vi "Grow primitive into new lattice vectors.vi"(6 "Max # of atoms":i32=9999999, 7 "Keep old lattice vectors?":bool, 8 "New Lattice Vector c":dbl[](array[numeric])=[0.0, 0.0, 6.0], 9 "New Lattice Vector b":dbl[](array[numeric])=[0.0, 6.0, 0.0], 10 "New Lattice Vector a":dbl[](array[numeric])=[6.0, 0.0, 0.0], 11 "Primitive":T1={"Structure Name"="Gamm8 Subcrystal", "Lattice vector a"=[2.3379684769090283, 4.050155798593294, -3.073453095936429e-05], "Lattice vector b"=[0.0, 2.7000749366574968, 3.8175198422845327], "Lattice vector c"=[4.675927601962877, 0.0, 0.0], "Atoms Array"=[{"Atom Name"="Cd", "Positions (Direct)"=[[0.0, 2.2797955771e-06, 0.2499966378910753]], "Positions (Cartesian)"=[[0.0, -3.2294507389786483e-06, 2.863111017657439]]}, {"Atom Name"="Te", "Positions (Direct)"=[[0.0, -2.2797955771e-06, 3.3621089247e-06]], "Positions (Cartesian)"=[[0.0, -1.5237858666867705e-05, -2.8630725126350507]]}], "# of atoms"=2} {"Atoms Array"."Positions (Cartesian)" format="%#_4f"; "Atoms Array"."Positions (Direct)" format="%#_4f"}) -> (0 "error out":errorcluster, 2 "Supercells Filled":dbl[][](array[numeric]), 3 "Expanded to new Vectors":T1={"Structure Name"="Gamm8 Subcrystal", "Lattice vector a"=[2.3379684769090283, 4.050155798593294, -3.073453095936429e-05], "Lattice vector b"=[0.0, 2.7000749366574968, 3.8175198422845327], "Lattice vector c"=[4.675927601962877, 0.0, 0.0], "Atoms Array"=[{"Atom Name"="Cd", "Positions (Direct)"=[[0.0, 2.2797955771e-06, 0.2499966378910753]], "Positions (Cartesian)"=[[0.0, -3.2294507389786483e-06, 2.863111017657439]]}, {"Atom Name"="Te", "Positions (Direct)"=[[0.0, -2.2797955771e-06, 3.3621089247e-06]], "Positions (Cartesian)"=[[0.0, -1.5237858666867705e-05, -2.8630725126350507]]}], "# of atoms"=2} {"Atoms Array"."Positions (Cartesian)" format="%#_4f"; "Atoms Array"."Positions (Direct)" format="%#_4f"})   [LabVIEW 2010]
uses:
  <vilib>/Analysis/baseanly.llb/Real Inverse Matrix.vi
  <vilib>/Analysis/baseanly.llb/A x Vector.vi
  <vilib>/Analysis/NI_AALBase.lvlib
panel:
  out "Numeric 2":i32
  out "Numeric":i32
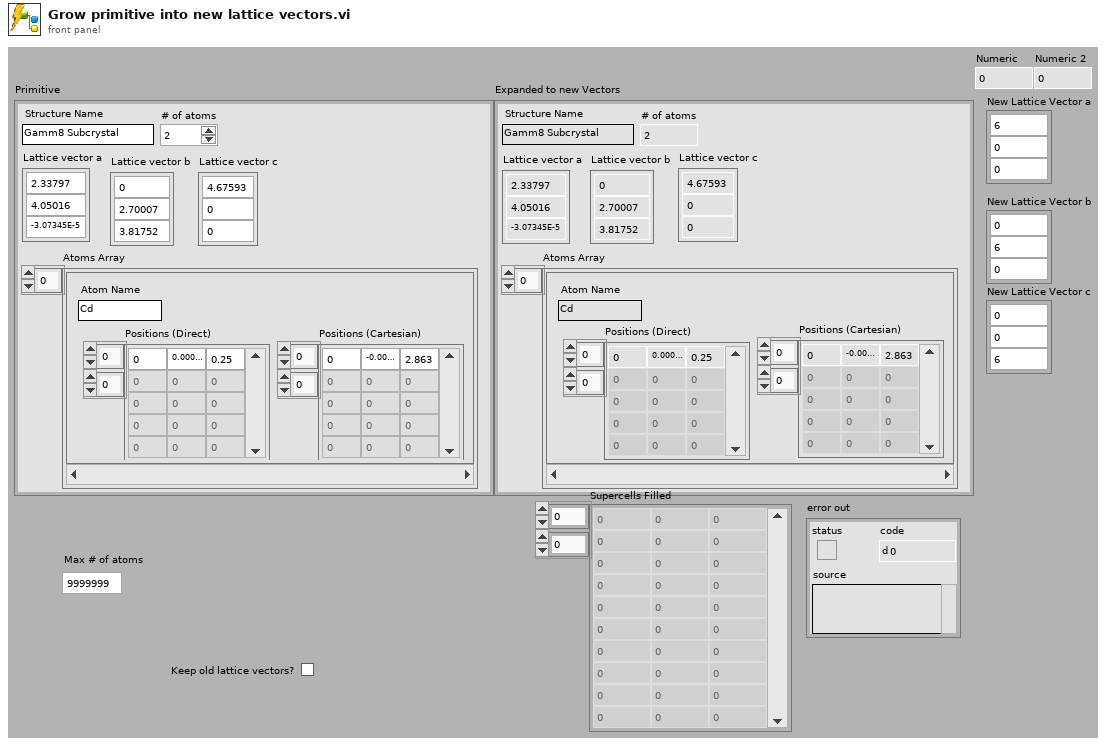
[diagram p1: front panel]
types:
  T1 = cluster{"Structure Name":string, "Lattice vector a":dbl[], "Lattice vector b":dbl[], "Lattice vector c":dbl[], "Atoms Array":cluster{"Atom Name":string, "Positions (Direct)":dbl[][], "Positions (Cartesian)":dbl[][]}[], "# of atoms":i32}
  T2 = cluster{"Atom Name":string, "Positions (Direct)":dbl[][], "Positions (Cartesian)":dbl[][]}[]
  T3 = typedef "NI_Matrix.lvlib/RealMatrix.ctl" = dbl[][]
  T4 = cluster{"Atom Name":string, "Positions (Direct)":dbl[][], "Output Array":dbl[][]}
  T5 = cluster{string, "Lattice vector a":dbl[], "Lattice vector b":dbl[], "Lattice vector c":dbl[], cluster{"Atom Name":string, "Positions (Direct)":dbl[][], "Output Array":dbl[][]}[], i32}
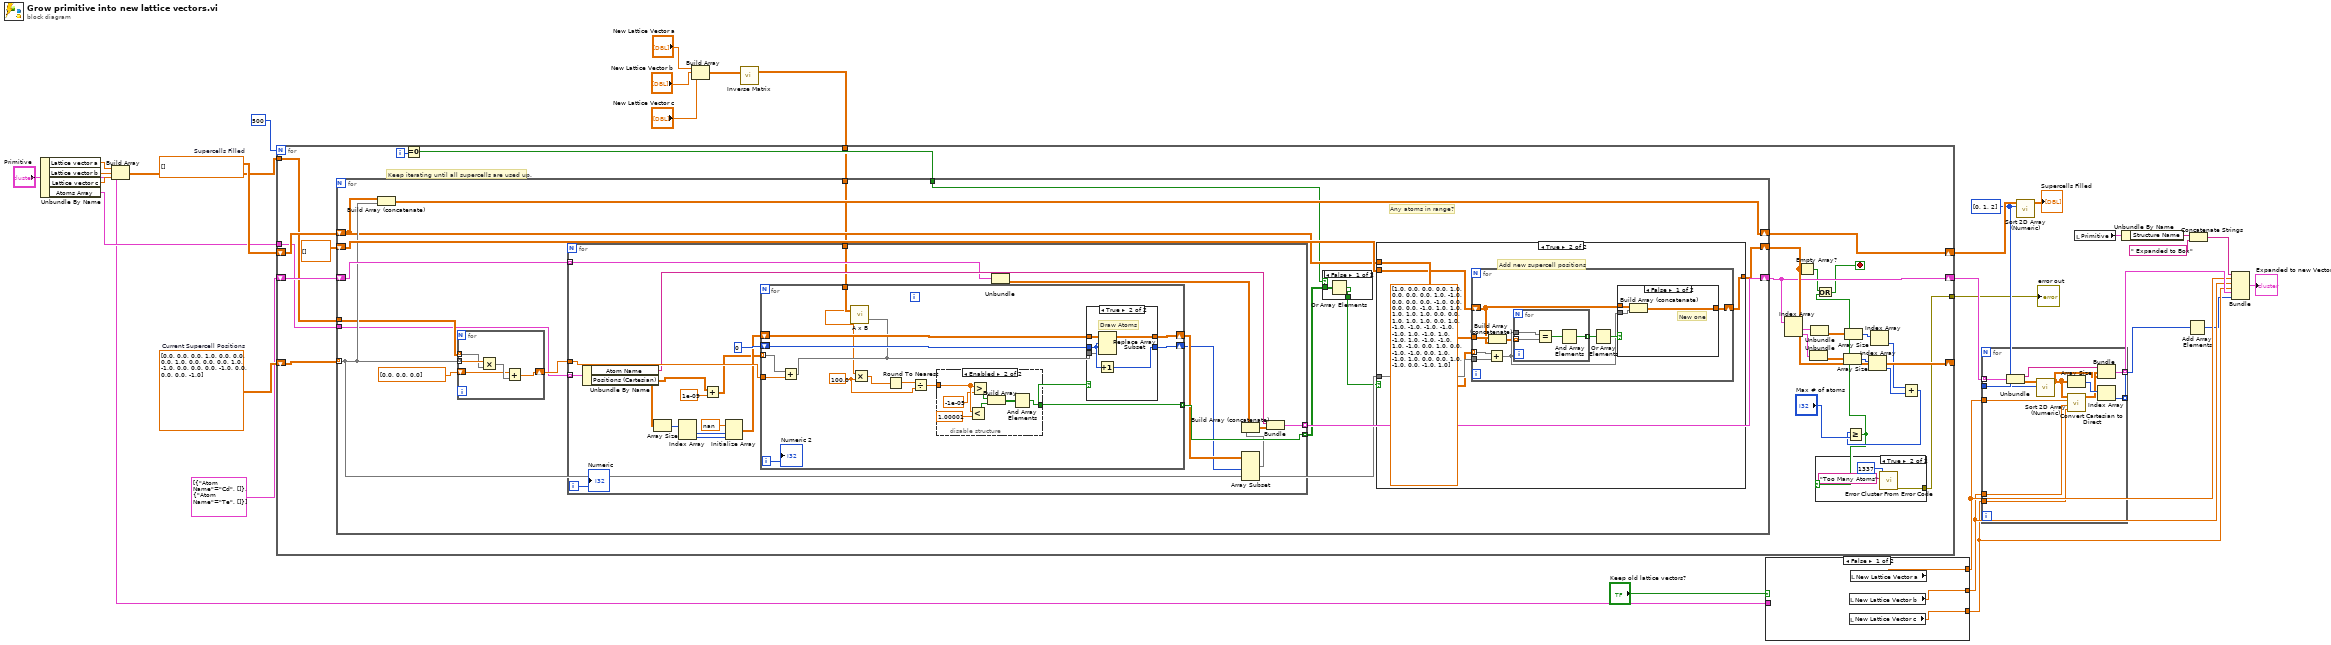
[diagram p0: block diagram]
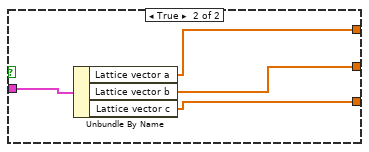
[diagram p2: hidden frame]
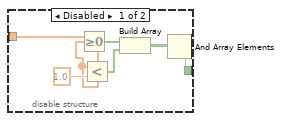
[diagram p7: hidden frame]
diagram:
  w20 = i32[] [0, 1, 2] ("Sort by Cols")
  w30 = dbl[][] []  # Supercells Filled
  w32 = dbl[][] [[0.0, 0.0, 0.0], [1.0, 0.0, 0.0], [0.0, 1.0, 0.0], [0.0, 0.0, 1.0], [-1.0, 0.0, 0.0], [0.0, -1.0, 0.0], [0.0, 0.0, -1.0]]  # Current Supercell Positions
  n1 = Unbundle By Name("Primitive") -> ("Lattice vector a"=w29:dbl[], "Lattice vector b"=w28:dbl[], "Lattice vector c"=w27:dbl[], "Atoms Array"=w25:T2)
  n2 = Build Array(w29, w28, w27) -> (w26:dbl[][])
  n3 = Build Array("New Lattice Vector a", "New Lattice Vector b", "New Lattice Vector c") -> (w2:T3)
  n4 = call-poly <vilib>:"Inverse Matrix.vi"("Input Matrix"=w2) -> ("Inverse Matrix"=w1:T3)  [unwired: 1 in, 1 out]
  n5 = for {
    N: 500 -> [_]
    shift-right: [w52] -> _
    shift-left: w32 -> [w33]
    shift-right: [w49] -> w21
    shift-left: cluster{"Atom Name":string, dbl[][]}[] [{"Atom Name"="Cd", []}, {"Atom Name"="Te", []}] -> [w57]
    shift-right: [w55] -> w24
    shift-left: w30 -> [w56]
    tunnel: w26 -> [w54]
    tunnel: w25 -> [w53]
    tunnel: [w35] -> w6
    tunnel: w1 -> [w34]
    i -> [w51]
    stop <- w44 stop-if-true
    # "Keep iterating until all supercells are used up."
    n6 = Equal To 0?(x=w51) -> (x = 0?=w50:bool)
    n7 = for {
      shift-right: [w71] -> w52
      shift-left: dbl[][] [] ("Supercell Positions") -> [w74]
      tunnel: w33 -> [w70] mode=indexing
      shift-right: [w73] -> w49
      shift-left: w57 -> [w72]
      shift-right: [w66] -> w55
      shift-left: w56 -> [w69]
      tunnel: w54 -> [w68]
      tunnel: w53 -> [w67]
      tunnel: w50 -> [w63]
      tunnel: w34 -> [w62]
      # "Any atoms in range?"
      n8 = Build Array (concatenate)(w69, w70) -> (w66:dbl[][])
      n9 = for {
        tunnel: w70 -> [w107] mode=indexing
        shift-right: [w105] -> w75
        shift-left: dbl[] [0.0, 0.0, 0.0] -> [w104]
        tunnel: w68 -> [w103] mode=indexing
        n10 = Multiply(x=w107, y=w103) -> (x*y=w106:dbl[])
        n11 = Add(x=w104, y=w106) -> (x+y=w105:dbl[])
      }
      n12 = for {
        tunnel: w67 -> [w128] mode=indexing
        tunnel: w75 -> [w129]
        tunnel: [w127] -> w65 mode=indexing
        tunnel: w72 -> [w124] mode=indexing
        tunnel: [w125] -> w73 mode=indexing
        tunnel: w62 -> [w112]
        i -> [w108]
        n13 = Unbundle By Name(w128) -> ("Atom Name"=w126:string, "Positions (Cartesian)"=w110:dbl[][])
        n14 = Array Size(array=w110) -> (size(s)=w118:i32[])
        n15 = Index Array(array=w118) -> (element #1=w117:i32, element #2=w116:i32)  [unwired: 2 in]
        n16 = Add(x=w110, y=1e-09) -> (x+y=w109:dbl[][])
        n17 = Initialize Array(nan ("element"), w117, w116) -> (w119:dbl[][])
        n18 = for {
          tunnel: w109 -> [w144] mode=indexing
          tunnel: w129 -> [w143]
          shift-right: [w142] -> w115
          shift-left: w119 -> [w141]
          tunnel: [w137] -> w127 mode=indexing
          shift-right: [w139] -> w114
          shift-left: 0 -> [w140]
          tunnel: w112 -> [w138]
          i -> [w133]
          w134 = 100.0 ("y")
          n19 = Add(x=w144, y=w143) -> (x+y=w132:dbl[])
          n20 = call-poly <vilib>:"A x B.vi"("Vector"=w132, "A"=w138) -> ("A x Vector"=w131:dbl[])  [unwired: 1 out]
          n21 = Multiply(x=w131, y=w134) -> (x*y=w136:dbl[])
          n22 = Round To Nearest(number=w136) -> (nearest integer value=w135:dbl[])
          n23 = Divide(x=w135, y=w134) -> (x/y=w130:dbl[])
          n24 = disable-structure shown="Enabled" {
            disable-tunnel: [w146 w152] -> w137
            disable-tunnel: w130 -> [w145 w156]
            frame Disabled {
              n25 = Greater Or Equal To 0?(x=w145) -> (x >= 0?=w149:bool[])
              n26 = Less?(x=w145, y=1.0) -> (x < y?=w148:bool[])
              n27 = Build Array(w149, w148) -> (w147:bool[][])
              n28 = And Array Elements(Boolean array=w147) -> (logical AND=w146:bool)
            }
            frame Enabled {
              n29 = Less?(x=w156, y=1.00001) -> (x < y?=w154:bool[])
              n30 = Greater?(x=w156, y=-1e-05) -> (0:w153:bool[])
              n31 = Build Array(w153, w154) -> (w155:bool[][])
              n32 = And Array Elements(Boolean array=w155) -> (logical AND=w152:bool)
            }
          }
          n33 = case shown="True" w137 {
            tunnel: w132 -> [_ w161]
            tunnel: [w159 w160] -> w142
            tunnel: w141 -> [w159 w163]
            tunnel: w140 -> [w158 w162]
            tunnel: [w158 w164] -> w139
            frame False {
              # "Not inside box"
            }
            frame True {
              # "Draw Atoms"
              n34 = Increment(x=w162) -> (x+1=w164:i32)
              n35 = Replace Array Subset(array=w163, new element=w161, index (row)=w162) -> (w160:dbl[][])  [unwired: 1 in]
            }
          }
          "Numeric 2" <- w133
        }
        n36 = Unbundle(w124) -> (w122:dbl[][])  [unwired: 1 out]
        n37 = Array Subset(array=w115, length (row)=w114) -> (w113:dbl[][])  [unwired: 3 in]
        n38 = Build Array (concatenate)(w122, w113) -> (w121:dbl[][])
        n39 = Bundle("Atom Name"=w126, w121) -> (w125:cluster{"Atom Name":string, dbl[][]})  [unwired: 1 in]
        "Numeric" <- w108
      }
      n40 = case shown="False" w63 {
        selector: w63 -> [_ w79]
        tunnel: w65 -> [w78 _]
        tunnel: [w77 w79] -> w64
        frame False {
          n41 = Or Array Elements(Boolean array=w78) -> (logical OR=w77:bool)
        }
        frame True {
        }
      }
      n42 = case shown="True" w64 {
        tunnel: w70 -> [_ w85]
        tunnel: [w80 w81] -> w71
        tunnel: w74 -> [w80 w82]
        tunnel: w69 -> [_ w83]
        frame False {
          # "Don't sweat it"
        }
        frame True {
          # "Add new supercell positions"
          n43 = for {
            tunnel: w85 -> [w93]
            tunnel: dbl[][] [[1.0, 0.0, 0.0], [0.0, 1.0, 0.0], [0.0, 0.0, 1.0], [-1.0, 0.0, 0.0], [0.0, -1.0, 0.0], [0.0, 0.0, -1.0], [1.0, 1.0, 1.0], [1.0, 1.0, 0.0], [0.0, 1.0, 1.0], [1.0, 0.0, 1.0], [-1.0, -1.0, -1.0], [-1.0, -1.0, 1.0], [-1.0, 1.0, -1.0], [1.0, -1.0, -1.0], [1.0, -1.0, 0.0], [1.0, 0.0, -1.0], [-1.0, 0.0, 1.0], [-1.0, 1.0, 0.0], [0.0, 1.0, -1.0], [0.0, -1.0, 1.0]] -> [w94] mode=indexing
            tunnel: w83 -> [w88]
            shift-right: [w92] -> w81
            shift-left: w82 -> [w87]
            n44 = Add(x=w94, y=w93) -> (x+y=w90:dbl[])
            n45 = Build Array (concatenate)(w88, w87) -> (w86:dbl[][])
            n46 = for {
              tunnel: w90 -> [w102]
              tunnel: w86 -> [w101] mode=indexing
              tunnel: [w99] -> w89 mode=indexing
              n47 = Equal?(x=w102, y=w101) -> (x = y?=w100:bool[])
              n48 = And Array Elements(Boolean array=w100) -> (logical AND=w99:bool)
            }
            n49 = Or Array Elements(Boolean array=w89) -> (logical OR=w91:bool)
            n50 = case shown="False" w91 {
              tunnel: w90 -> [w97 _]
              tunnel: [w96 w98] -> w92
              tunnel: w87 -> [w95 w98]
              frame False {
                # "New one"
                n51 = Build Array (concatenate)(w95, w97) -> (w96:dbl[][])
              }
              frame True {
                # "Already Did this one"
              }
            }
          }
        }
      }
    }
    n52 = Index Array(array=w49) -> (element #1=w48:cluster{"Atom Name":string, dbl[][]}, element #2=w40:cluster{"Atom Name":string, dbl[][]})  [unwired: 2 in]
    n53 = Empty Array?(array=w52) -> (empty?=w45:bool)
    n54 = Unbundle(w40) -> (w41:dbl[][])  [unwired: 1 out]
    n55 = Unbundle(w48) -> (w47:dbl[][])  [unwired: 1 out]
    n56 = Array Size(array=w41) -> (size(s)=w42:i32[])
    n57 = Array Size(array=w47) -> (size(s)=w46:i32[])
    n58 = Index Array(array=w42) -> (element=w38:i32)  [unwired: 1 in]
    n59 = Index Array(array=w46) -> (element=w39:i32)  [unwired: 1 in]
    n60 = Add(x=w39, y=w38) -> (x+y=w37:i32)
    n61 = Greater Or Equal?(x=w37, y="Max # of atoms") -> (x >= y?=w36:bool)
    n62 = case shown="True" w36 {
      tunnel: [_ w61] -> w35
      frame False {
      }
      frame True {
        n63 = call <vilib>:"Error Cluster From Error Code.vi"("error message (\"\")"="Too Many Atoms" ("error message (\"\")"), "error code (0)"=1337) -> ("error out"=w61:errorcluster)  [unwired: 7 in]
      }
    }
    n64 = Or(x=w45, y=w36) -> (x .or. y?=w44:bool)
  }
  "error out" <- w6
  n65 = case shown="False" "Keep old lattice vectors?" {
    tunnel: [w167 w170] -> w18
    tunnel: [w165 w169] -> w17
    tunnel: [w166 w168] -> w16
    tunnel: "Primitive" -> [_ w171]
    frame False {
      n66 = local read "New Lattice Vector b"() -> (w165:dbl[])
      n67 = local read "New Lattice Vector c"() -> (w166:dbl[])
      n68 = local read "New Lattice Vector a"() -> (w167:dbl[])
    }
    frame True {
      n69 = Unbundle By Name(w171) -> ("Lattice vector a"=w170:dbl[], "Lattice vector b"=w169:dbl[], "Lattice vector c"=w168:dbl[])
    }
  }
  n70 = for {
    tunnel: w21 -> [w183] mode=indexing
    tunnel: w20 -> [w181]
    tunnel: [w179] -> w19 mode=indexing
    tunnel: w18 -> [w178]
    tunnel: w17 -> [w177]
    tunnel: w16 -> [w176]
    tunnel: [w174] -> w11 mode=indexing
    n71 = Unbundle(w183) -> ("Atom Name"=w180:string, w182:dbl[][])
    n72 = call "Sort 2D Array (Numeric).vi"("Sort by Cols"=w181, "Input Array"=w182) -> ("Output Array"=w172:dbl[][])  [unwired: 9 in]
    n73 = Array Size(array=w172) -> (size(s)=w175:i32[])
    n74 = call "Convert Cartesian to Direct.vi"("Lattice vector c"=w176, "Lattice vector b"=w177, "Lattice vector a"=w178, "Positions (Cartesian)"=w172) -> ("Positions (Direct)"=w173:dbl[][])  [unwired: 7 in]
    n75 = Bundle("Atom Name"=w180, "Positions (Direct)"=w173, "Output Array"=w172) -> (w179:T4)  [unwired: 1 in]
    n76 = Index Array(array=w175) -> (element=w174:i32)  [unwired: 1 in]
  }
  n77 = call "Sort 2D Array (Numeric).vi"("Sort by Cols"=w20, "Input Array"=w24) -> ("Output Array"=→"Supercells Filled":dbl[][])  [unwired: 9 in]
  n78 = local read "Primitive"() -> (w15:T1)
  n79 = Unbundle By Name(w15) -> ("Structure Name"=w14:string)
  n80 = Add Array Elements(numeric array=w11) -> (sum=w10:i32)
  n81 = Concatenate Strings(w14, " Expanded to Box" ("string")) -> (w12:string)
  n82 = Bundle(w12, "Lattice vector a"=w18, "Lattice vector b"=w17, "Lattice vector c"=w16, w19, w10) -> (→"Expanded to new Vectors":T5)  [unwired: 1 in]
